vi "CLSUIP_ArrangeFPTerms.vi"(8 "error in (no error)":errorcluster, 10 "Terminals as icons":bool, 11 "Node Refnum":refnum<vi>) -> (0 "error out":errorcluster)   [LabVIEW 2021, in "MemberVICreation.lvlib"]
uses:
  <resource>/Framework/Providers/LVClassLibrary/NewAccessors/MemberVICreation.lvlib
  <resource>/Framework/Providers/LVClassLibrary/NewAccessors/VIRetooler/VIRetooler.lvclass
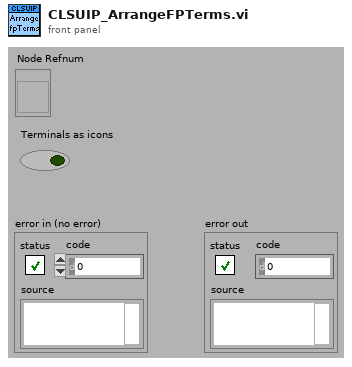
[diagram p1: front panel]
types:
  T1 = typedef "LVRectTypeDef.ctl" = cluster{"left":i16, "top":i16, "right":i16, "bottom":i16}
  T2 = cluster{"left":i16, "top":i16, "right":i16, "bottom":i16}
  T3 = cluster{"left":i16, "top":i16, "right":i16, "bottom":i16}[]
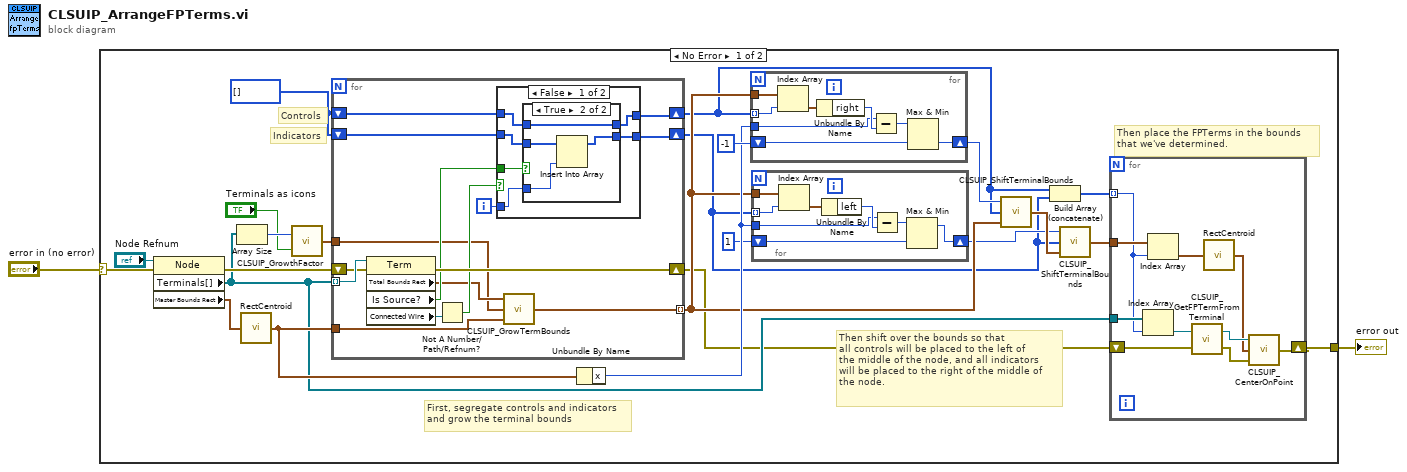
[diagram p0: block diagram]
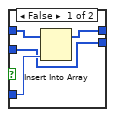
[diagram p2: hidden frame]
diagram:
  n1 = case shown="No Error" "error in (no error)" {
    selector: "error in (no error)" -> [w23 w83]
    tunnel: [w5 w83] -> w1
    frame No Error {
      w19 = i32[] []
      # "Then place the FPTerms in the bounds\nthat we've determined."
      # "Then shift over the bounds so that\nall controls will be placed to the left of \nthe middle of the node, and all indicators\nwill be placed to the right of the middle of\nthe node."
      # "First, segregate controls and indicators\nand grow the terminal bounds"
      # "Indicators"
      # "Controls"
      n2 = property class="Node"(reference="Node Refnum", error in=w23) -> (error out=w24:errorcluster, "Terminals[]"=w7:refnum<vi>[], "Master Bounds Rect"=w4:T1)  [unwired: 1 out]
      n3 = Array Size(array=w7) -> (size(s)=w22:i32)
      n4 = call <vilib>:"RectCentroid.vi"("rect"=w4) -> ("point"=w18:cluster{"x":i16, "y":i16})
      n5 = call <resource>:"CLSUIP_GrowthFactor.vi"("Terminals as icons"="Terminals as icons", "Number of terminals"=w22) -> ("Multiplication Factor"=w20:cluster{"Left":i32, "Top":i32})
      n6 = for {
        tunnel: w7 -> [w66] mode=indexing
        shift-right: [w64] -> w6
        shift-left: w24 -> [w65]
        tunnel: w18 -> [w53]
        tunnel: w20 -> [w54]
        shift-right: [w57] -> w11
        shift-left: w19 -> [w60]
        shift-right: [w56] -> w10
        shift-left: w19 -> [w59]
        tunnel: [w52] -> w15 mode=indexing
        i -> [w58]
        n7 = property class="Term"(reference=w66, error in=w65) -> (error out=w64:errorcluster, "Total Bounds Rect"=w55:T1, "Is Source?"=w61:bool, "Connected Wire"=w63:refnum<vi>)  [unwired: 1 out]
        n8 = Not A Number/Path/Refnum?(number/path/refnum=w63) -> (NaN/Path/Refnum?=w62:bool)
        n9 = case shown="False" w62 {
          tunnel: w61 -> [w72 _]
          tunnel: w60 -> [w68 w82]
          tunnel: w59 -> [w70 w81]
          tunnel: w58 -> [w71 _]
          tunnel: [w69 w82] -> w57
          tunnel: [w67 w81] -> w56
          frame False {
            n10 = case shown="True" w72 {
              tunnel: w71 -> [w74 w77]
              tunnel: w70 -> [w73 w80]
              tunnel: [w75 w79] -> w69
              tunnel: w68 -> [w76 w79]
              tunnel: [w73 w78] -> w67
              frame False {
                n11 = Insert Into Array(array=w76, new element=w74) -> (w75:i32[])  [unwired: 1 in]
              }
              frame True {
                n12 = Insert Into Array(array=w80, new element=w77) -> (w78:i32[])  [unwired: 1 in]
              }
            }
          }
          frame True {
          }
        }
        n13 = call <resource>:"CLSUIP_GrowTermBounds.vi"("Center Point"=w53, "Multiplication Factor"=w54, "Terminal Bounds"=w55) -> ("Grown Bounds"=w52:T2)
      }
      n14 = Unbundle By Name(w18) -> ("x"=w16:i16)
      n15 = for {
        tunnel: w11 -> [w50] mode=indexing
        tunnel: w15 -> [w51]
        tunnel: w16 -> [w47]
        shift-right: [w44] -> w14
        shift-left: -1 -> [w45]
        n16 = Index Array(array=w51, index=w50) -> (element=w49:T2)
        n17 = Unbundle By Name(w49) -> ("right"=w48:i16)
        n18 = Subtract(x=w47, y=w48) -> (x-y=w46:i16)
        n19 = Max & Min(x=w46, y=w45) -> (min(x,y)=w44:i32)  [unwired: 1 out]
      }
      n20 = for {
        tunnel: w10 -> [w42] mode=indexing
        tunnel: w15 -> [w43]
        tunnel: w16 -> [w39]
        shift-right: [w36] -> w12
        shift-left: 1 -> [w37]
        n21 = Index Array(array=w43, index=w42) -> (element=w41:T2)
        n22 = Unbundle By Name(w41) -> ("left"=w40:i16)
        n23 = Subtract(x=w39, y=w40) -> (x-y=w38:i16)
        n24 = Max & Min(x=w38, y=w37) -> (max(x,y)=w36:i32)  [unwired: 1 out]
      }
      n25 = call <resource>:"CLSUIP_ShiftTerminalBounds.vi"("Terminal Bounds"=w15, "Indices"=w11, "Shift Amount"=w14) -> ("Terminal Bounds out"=w13:T3)
      n26 = Build Array (concatenate)(w11, w10) -> (w9:i32[])
      n27 = call <resource>:"CLSUIP_ShiftTerminalBounds.vi"("Terminal Bounds"=w13, "Indices"=w10, "Shift Amount"=w12) -> ("Terminal Bounds out"=w8:T3)
      n28 = for {
        tunnel: w9 -> [w29] mode=indexing
        tunnel: w8 -> [w30]
        tunnel: w7 -> [w34]
        shift-right: [w27] -> w5
        shift-left: w6 -> [w35]
        n29 = Index Array(array=w34, index=w29) -> (element=w33:refnum<vi>)
        n30 = Index Array(array=w30, index=w29) -> (element=w28:T2)
        n31 = call <resource>:"CLSUIP_GetFPTermFromTerminal.vi"("error in (no error)"=w35, "Term Refnum"=w33) -> ("error out"=w31:errorcluster, "CtrlTerm Refnum"=w32:refnum<vi>)
        n32 = call <vilib>:"RectCentroid.vi"("rect"=w28) -> ("point"=w26:cluster{"x":i16, "y":i16})
        n33 = call <resource>:"CLSUIP_CenterOnPoint.vi"("error in (no error)"=w31, "Position"=w26, "CtrlTerm Refnum"=w32) -> ("error out"=w27:errorcluster)
      }
    }
    frame Error {
    }
  }
  "error out" <- w1
